vi "Clousure.vi"(8 "error in (no error)":errorcluster, 11 "Room":refnum<class "Room.lvclass">) -> (0 "error out":errorcluster, 3 "Room":refnum<class "Room.lvclass">)   [LabVIEW 2020, in "Room.lvclass"]
uses:
  Room.lvclass
  Room.lvclass/Room.ctl
  Private/Property/side/Read side.vi
  MazeSite/MazeSite.lvclass
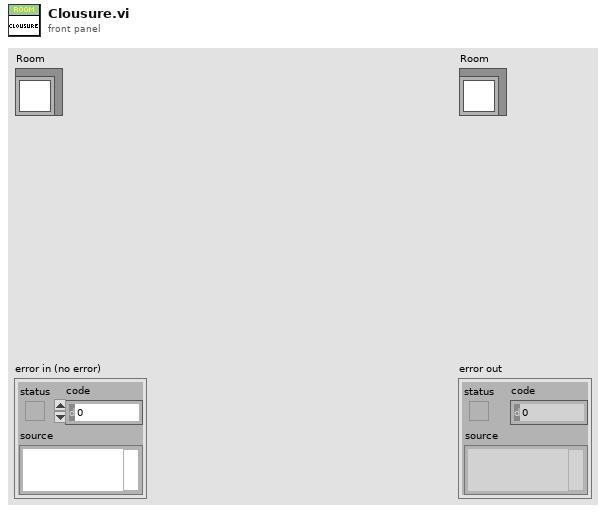
[diagram p1: front panel]
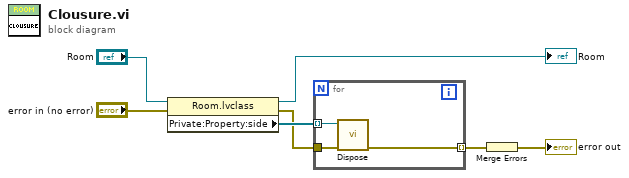
[diagram p0: block diagram]
diagram:
  n1 = property class="Room.lvclass"(reference="Room", error in="error in (no error)") -> (reference out=→"Room":refnum<class "Room.lvclass">, error out=w5:errorcluster, "Private:Property:side"=w6:refnum<class "MazeSite.lvclass">[])
  n2 = for {
    tunnel: w6 -> [w10] mode=indexing
    tunnel: w5 -> [w9]
    tunnel: [w8] -> w4 mode=indexing
    n3 = call-dynamic "Dispose.vi"("error in (no error)"=w9, "IDisposable"=w10) -> ("error out"=w8:errorcluster)  [unwired: 9 in]
  }
  n4 = Merge Errors(w4) -> (→"error out":errorcluster)
